vi "GetBars.vi"(8 "error in (no error)":errorcluster, 10 "Munged Input":string, 11 "Code128 in":refnum<class "Code128.lvclass">) -> (0 "error out":errorcluster, 2 "BarWidths":T1[][](array[typedef]), 3 "Code128 out":refnum<class "Code128.lvclass">)   [LabVIEW 2013, in "BarCodes.lvlib" / "Code128.lvclass"]
doc: "Gets the bars of the bar code. The bars are specified as an array of bar widths from left to right."
uses:
  Code128.lvclass
  BarCode/Bar.ctl
  Code128.lvclass/Code128.ctl
  BarCode/BarCode.lvclass
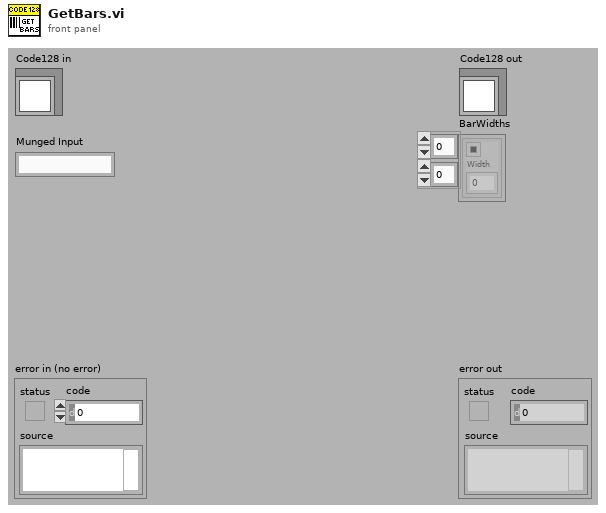
[diagram p1: front panel]
types:
  T1 = typedef "BarCodes.lvlib/BarCode.lvclass/Bar.ctl" = cluster{"Color":u32, "Width":u8}
  T2 = typedef "BarCodes.lvlib/Code128.lvclass/CharacterInfo.ctl" = cluster{"Character":string, "Bars":u8[]}
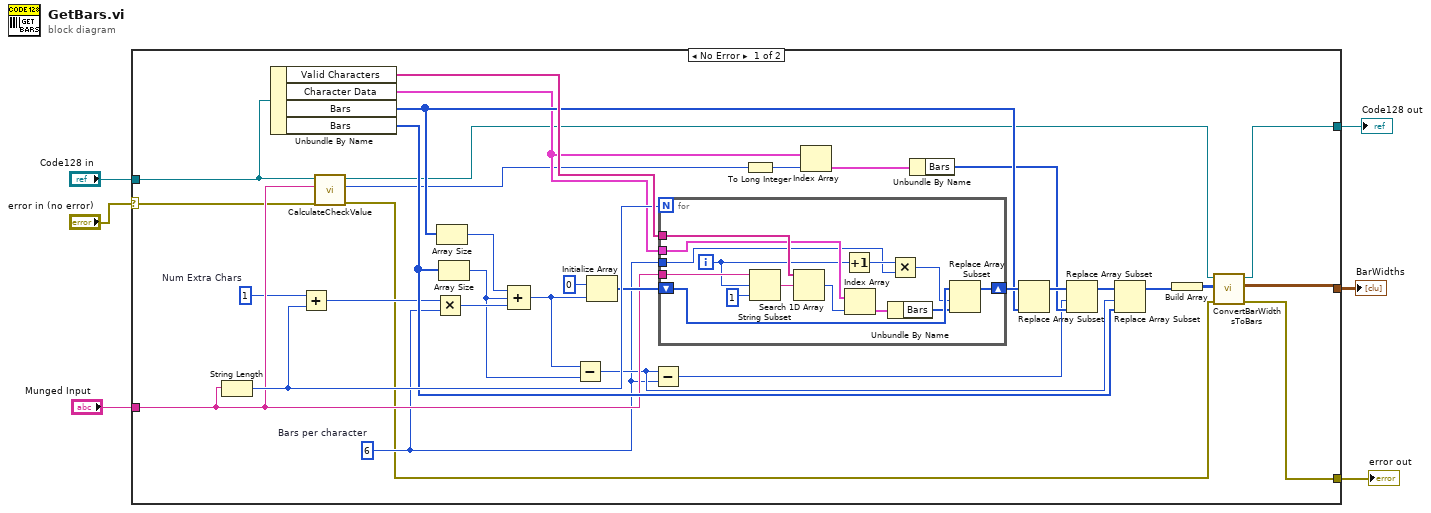
[diagram p0: block diagram]
diagram:
  n1 = case shown="No Error" "error in (no error)" {
    selector: "error in (no error)" -> [w15 w54]
    tunnel: "Code128 in" -> [w29 w55]
    tunnel: [w10 w55] -> w5
    tunnel: [w8 w54] -> w4
    tunnel: "Munged Input" -> [w28 _]
    tunnel: [w9 _] -> w1
    frame No Error {
      w23 = 1  # Num Extra Chars
      w18 = 6  # Bars per character
      n2 = String Length(string=w28) -> (length=w38:i32)
      n3 = Unbundle By Name(w29) -> ("Valid Characters"=w39:string[], "Character Data"=w27:T2[], "Bars"=w34:u8[], "Bars"=w33:u8[])
      n4 = Add(x=w23, y=w38) -> (x+y=w32:i32)
      n5 = call "CalculateCheckValue.vi"("error in (no error)"=w15, "String"=w28, "Code128 in"=w29) -> ("error out"=w7:errorcluster, "Numeric"=w26:u8, "Code128 out"=w11:refnum<class "Code128.lvclass">)  [unwired: 6 in]
      n6 = Multiply(x=w32, y=w18) -> (x*y=w21:i32)
      n7 = Array Size(array=w34) -> (size(s)=w22:i32)
      n8 = Array Size(array=w33) -> (size(s)=w20:i32)
      n9 = Compound Arithmetic op=ADD(w22, w20, w21) -> (w16:i32)
      n10 = Subtract(x=w16, y=w20) -> (x-y=w19:i32)
      n11 = Initialize Array(u8 0 ("Numeric"), w16) -> (w36:u8[])
      n12 = Subtract(x=w19, y=w18) -> (x-y=w17:i32)
      n13 = for {
        N: w38 -> [_]
        tunnel: w28 -> [w53]
        tunnel: w39 -> [w51]
        tunnel: w27 -> [w49]
        shift-right: [w45] -> w35
        shift-left: w36 -> [w47]
        tunnel: w18 -> [w40]
        i -> [w42]
        n14 = String Subset(string=w53, offset (0)=w42, length (rest)=1 ("length (rest)")) -> (substring=w50:string)
        n15 = Search 1D Array(1D array=w51, element=w50) -> (index of element=w48:i32)  [unwired: 1 in]
        n16 = Increment(x=w42) -> (x+1=w41:i32)
        n17 = Index Array(array=w49, index=w48) -> (element=w44:T2)
        n18 = Unbundle By Name(w44) -> ("Bars"=w43:u8[])
        n19 = Multiply(x=w41, y=w40) -> (x*y=w46:i32)
        n20 = Replace Array Subset(array=w47, new element=w43, index=w46) -> (w45:u8[])
      }
      n21 = To Long Integer(number=w26) -> (32bit integer=w14:i32)
      n22 = Index Array(array=w27, index=w14) -> (element=w25:T2)
      n23 = Unbundle By Name(w25) -> ("Bars"=w24:u8[])
      n24 = Replace Array Subset(array=w35, new element=w34) -> (w31:u8[])  [unwired: 1 in]
      n25 = Replace Array Subset(array=w31, new element=w24, index=w17) -> (w30:u8[])
      n26 = Replace Array Subset(array=w30, new element=w33, index=w19) -> (w13:u8[])
      n27 = Build Array(w13) -> (w12:u8[][])
      n28 = call "ConvertBarWidthsToBars.vi"("error in (no error)"=w7, "BarWidths"=w12, "BarCode in"=w11) -> ("error out"=w8:errorcluster, "Bars"=w9:T1[][], "BarCode out"=w10:refnum<class "Code128.lvclass">)  [unwired: 6 in]
    }
    frame Error {
    }
  }
  "error out" <- w4
  "Code128 out" <- w5
  "BarWidths" <- w1
